vi "(Depricated) Sample In.vi"(8 "error in (no error)":errorcluster, 10 "Sample":refnum<class "Sample.lvclass">, 11 "Preparation Line in":refnum<class "Preparation Line.lvclass">=refnum) -> (0 "error out":errorcluster, 3 "Preparation Line out":refnum<class "Preparation Line.lvclass">)   [LabVIEW 2015]
uses:
  Preparation Line.lvclass
  subs/Sample/Sample.lvclass
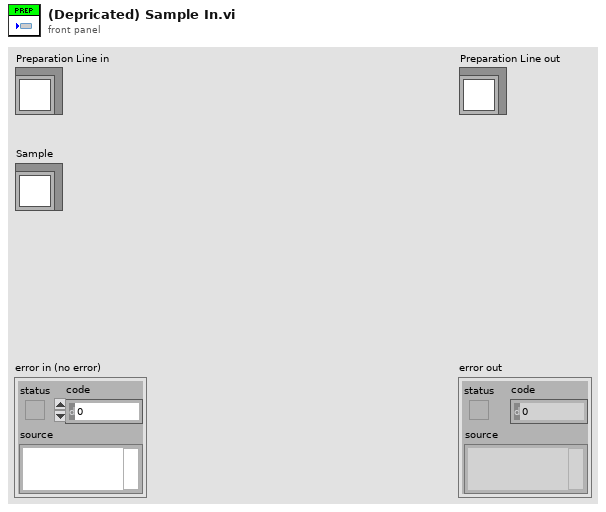
[diagram p1: front panel]
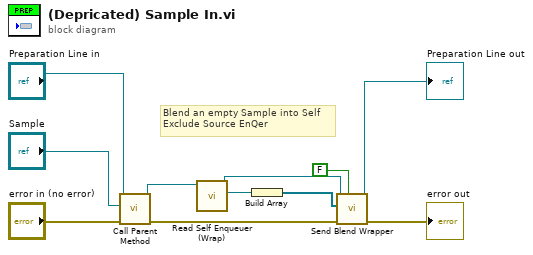
[diagram p0: block diagram]
diagram:
  # "Blend an empty Sample into Self\nExclude Source EnQer"
  n1 = call-parent "Call Parent Method"("error in (no error)"="error in (no error)", "Sample"="Sample", "CO2 Actor in"="Preparation Line in") -> ("error out"=w6:errorcluster, "CO2 Actor out"=w5:refnum<class "Preparation Line.lvclass">)  [unwired: 7 in]
  n2 = call "Read Self Enqueuer (Wrap).vi"("CO2 Actor in"=w5) -> ("Actor Framework:Message Enqueuer"=w3:refnum<class "Message Enqueuer.lvclass">, "CO2 Actor out"=w4:refnum<class "Preparation Line.lvclass">)  [unwired: 9 in]
  n3 = Build Array(w3) -> (w2:refnum<class "Message Enqueuer.lvclass">[])
  n4 = call-dynamic "Send Blend Wrapper.vi"("Include Source EnQr (T)"=FALSE, "error in (no error)"=w6, "Send to"=w2, "CO2 Actor in"=w4) -> ("error out"=→"error out":errorcluster, "CO2 Actor out"=→"Preparation Line out":refnum<class "Preparation Line.lvclass">)  [unwired: 6 in]
